vi "Test Match Pattern.vi"() -> ()   [LabVIEW 2020]
panel:
  out "match substring":string
  out "after substring":string
  in  "text 2":string
  out "text":string
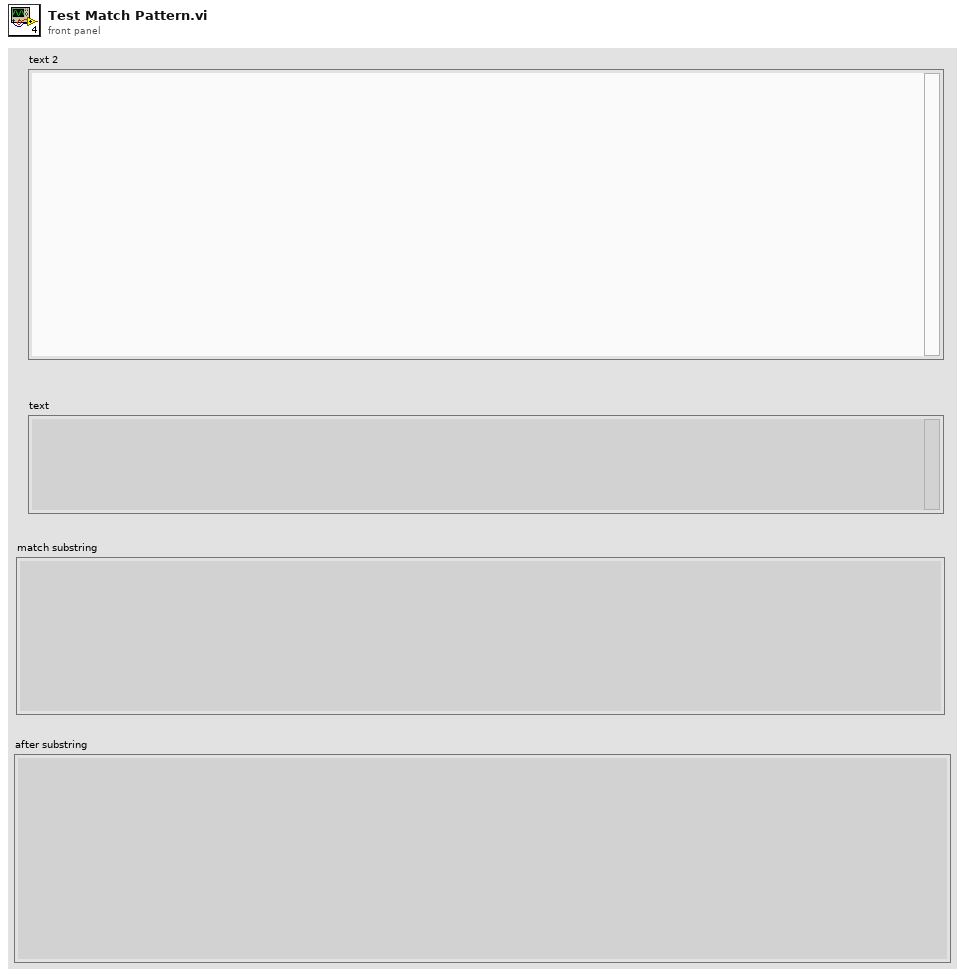
[diagram p1: front panel]
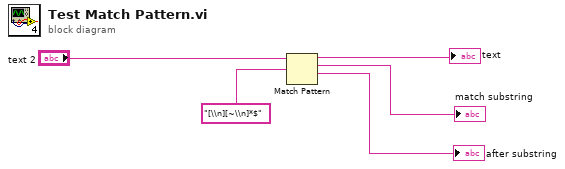
[diagram p0: block diagram]
diagram:
  n1 = Match Pattern(string="text 2", regular expression="[\\n][~\\n]*$") -> (before substring=→"text":string, match substring=→"match substring":string, after substring=→"after substring":string)  [unwired: 1 in, 1 out]
